vi "SimpleTriangleArea.vi"(1 "A":dbl, 2 "H":dbl) -> (0 "P":dbl)   [LabVIEW 2020]
doc: "Liczy pole z podstawowego wzoru korzystając z długości boku i wysokości na ten bok opadającej."
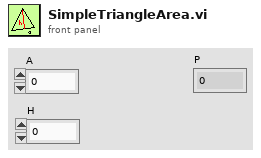
[diagram p1: front panel]
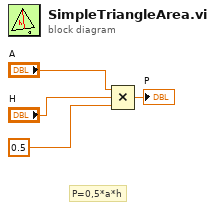
[diagram p0: block diagram]
diagram:
  # "P=0,5*a*h"
  n1 = Compound Arithmetic op=MULTIPLY("A", "H", 0.5 ("value")) -> (→"P":dbl)
